vi "Acquire and Log Data - Config .vi"(5 "FPGA VI Reference":T5, 7 "Total Buffer Size":i32, 8 "error in (no error)":errorcluster, 9 "Number of Blocks Saved in":i32, 10 "Acquisition Data v1":T1={"Data Rate"=1, "Samples per Read"=0, "Number of Reads to Save"=0, "Data File Name"="", "TDMS Properties"=[], "Number of Channels"=4, "Channel Scale Array"=[0.0, 0.0, 0.0, 0.0, 0.0, 0.0, 0.0, 0.0, 0.0, 0.0, 0.0, 0.0, 0.0, 0.0, 0.0, 0.0, 0.0, 0.0, 0.0, 0.0, 0.0, 0.0, 0.0, 0.0], "Channel Names"=[], "Trigger - RMS Value"=0.0, "Trigger - Channel"=0, "Trigger - Time (Minute)"=0, "Input Configuration"=0} {"Input Configuration" items=["AC Coupled", "DC Coupled", "IEPE AC Coupled"]; "Data Rate" items=["51.200 kS/s (NI 9234)"=1, "25.600 kS/s (NI 9234)"=2, "17.067 kS/s (NI 9234)"=3, "12.800 kS/s (NI 9234)"=4, "10.240 kS/s (NI 9234)"=5, "8.533 kS/s (NI 9234)"=6, "7.314 kS/s (NI 9234)"=7, "6.400 kS/s (NI 9234)"=8, "5.689 kS/s (NI 9234)"=9, "5.120 kS/s (NI 9234)"=10, "4.654 kS/s (NI 9234)"=11, "4.267 kS/s (NI 9234)"=12, "3.938 kS/s (NI 9234)"=13, "3.657 kS/s (NI 9234)"=14, "3.413 kS/s (NI 9234)"=15, "3.200 kS/s (NI 9234)"=16, "3.012 kS/s (NI 9234)"=17, "2.845 kS/s (NI 9234)"=18, "2.695 kS/s (NI 9234)"=19, "2.560 kS/s (NI 9234)"=20, "2.438 kS/s (NI 9234)"=21, "2.328 kS/s (NI 9234)"=22, "2.226 kS/s (NI 9234)"=23, "2.133 kS/s (NI 9234)"=24, "2.048 kS/s (NI 9234)"=25, "1.969 kS/s (NI 9234)"=26, "1.896 kS/s (NI 9234)"=27, "1.829 kS/s (NI 9234)"=28, "1.765 kS/s (NI 9234)"=29, "1.707 kS/s (NI 9234)"=30, "1.652 kS/s (NI 9234)"=31]}, 11 "TDMS File Reference":refnum<k34>) -> (0 "error out":errorcluster, 1 "Number of Blocks Saved out":i32, 3 "Logging Complete?":bool)   [LabVIEW 2015]
doc: "Reads waveform data from the DMA FIFO."
uses:
  controls/FPGA VI Reference.ctl
  controls/Acquisition and Logging Configuration_v1.ctl
  <vilib>/LabVIEW Targets/FPGA/cRIO/shared/nicrio_ModuleControls/nicrio_cRIO-9234_DataRatesRing2.ctl
  controls/TDMS Properties.ctl
  <vilib>/LabVIEW Targets/FPGA/cRIO/shared/nicrio_ModuleControls/nicrio_cRIO-9234_ConfigModeRing.ctl
  <vilib>/Analysis/5stat.llb/RMS (DBL).vi
  Globals/Global - Monitoring Variables.vi
  <vilib>/Analysis/NI_AALPro.lvlib
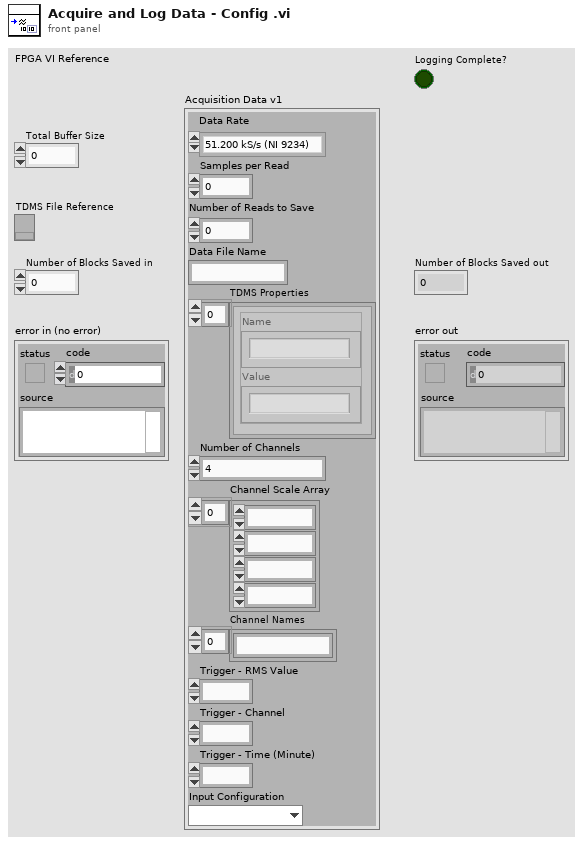
[diagram p1: front panel]
types:
  T1 = typedef "Acquisition and Logging Configuration_v1.ctl" = cluster{"Data Rate":T2, "Samples per Read":i32, "Number of Reads to Save":i32, "Data File Name":string, "TDMS Properties":T3[], "Number of Channels":i32, "Channel Scale Array":fxp<+,24,12>[], "Channel Names":string[], "Trigger - RMS Value":dbl, "Trigger - Channel":i32, "Trigger - Time (Minute)":i32, "Input Configuration":T4}
  T2 = typedef "nicrio_cRIO-9234_DataRatesRing2.ctl" = u8
  T3 = typedef "TDMS Properties.ctl" = cluster{"Name":string, "Value":string}
  T4 = typedef "nicrio_cRIO-9234_ConfigModeRing.ctl" = u8
  T5 = typedef "FPGA VI Reference.ctl" = refnum<k20>
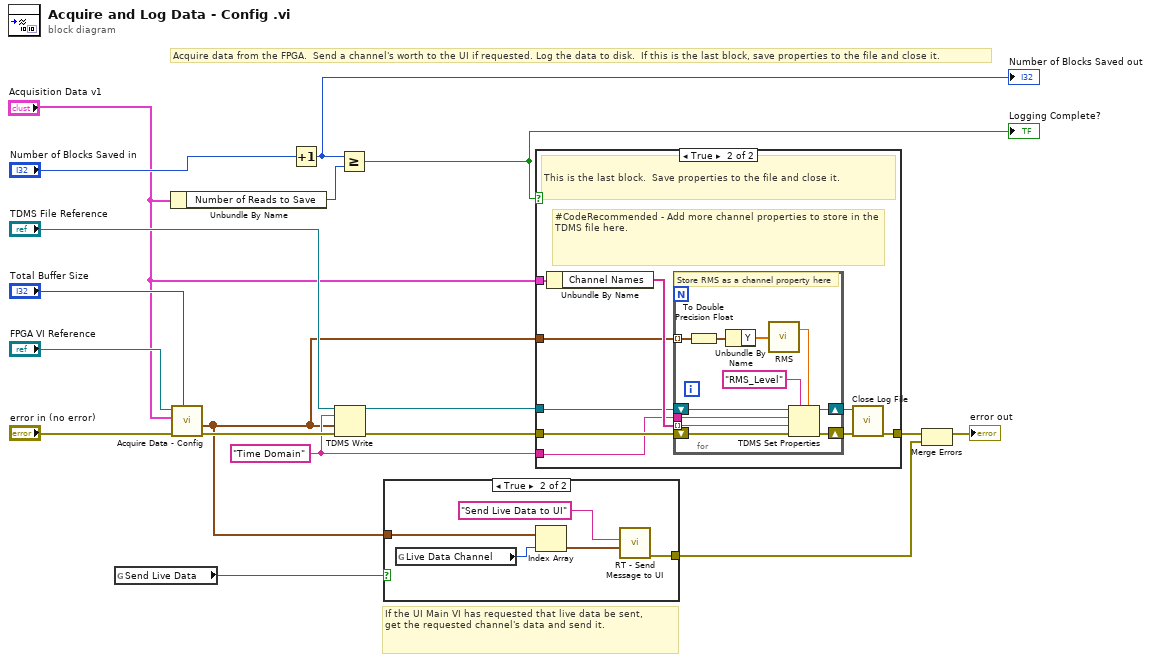
[diagram p0: block diagram]
diagram:
  w6 = "Time Domain" ("group name in (Untitled)")
  # "Acquire data from the FPGA.  Send a channel's worth to the UI if requested. Log the data to disk.  If this is the last block, save properties to the file and close it."
  # "If the UI Main VI has requested that live data be sent,\nget the requested channel's data and send it."
  n1 = global read "Global - Monitoring Variables.vi" "Send Live Data"() -> (w4:bool)
  n2 = Unbundle By Name("Acquisition Data v1") -> ("Number of Reads to Save"=w11:i32)
  n3 = call "Acquire Data - Config.vi"("Total Buffer Size"="Total Buffer Size", "error in (no error)"="error in (no error)", "Acquisition Data v1"="Acquisition Data v1", "FPGA VI Reference"="FPGA VI Reference") -> ("error out"=w15:errorcluster, "Waveform Data"=w3:waveform(sgl)[])  [unwired: 6 in]
  n4 = Increment(x="Number of Blocks Saved in") -> (x+1=w12:i32)
  "Number of Blocks Saved out" <- w12
  n5 = TDMS Write(0:"TDMS File Reference", 5:w6, 9:w3, 11:w15) -> (4:w9:refnum<k34>, 15:w8:errorcluster)  [unwired: 2 in, 2 out]
  n6 = Greater Or Equal?(x=w12, y=w11) -> (x >= y?=w10:bool)
  "Logging Complete?" <- w10
  n7 = case shown="True" w4 {
    tunnel: w3 -> [_ w23]
    tunnel: [_ w20] -> w2
    frame False {
    }
    frame True {
      n8 = global read "Global - Monitoring Variables.vi" "Live Data Channel"() -> (w22:u32)
      n9 = Index Array(array=w23, index=w22) -> (element=w21:waveform(sgl))
      n10 = call "RT - Send Message to UI.vi"("Message Data"=w21, "Message"="Send Live Data to UI" ("group name in (Untitled)")) -> ("error out"=w20:errorcluster)  [unwired: 9 in]
    }
  }
  n11 = case shown="True" w10 {
    tunnel: w9 -> [_ w29]
    tunnel: w8 -> [w24 w32]
    tunnel: [w24 w25] -> w7
    tunnel: "Acquisition Data v1" -> [_ w33]
    tunnel: w6 -> [_ w28]
    tunnel: w3 -> [_ w27]
    frame False {
      # "Do not finish the file.  This is not the last block."
    }
    frame True {
      # "#CodeRecommended - Add more channel properties to store in the TDMS file here."
      # "This is the last block.  Save properties to the file and close it."
      n12 = Unbundle By Name(w33) -> ("Channel Names"=w30:string[])
      n13 = for {
        tunnel: w28 -> [w41]
        shift-right: [w43] -> w31
        shift-left: w32 -> [w42]
        tunnel: w30 -> [w40] mode=indexing
        tunnel: w27 -> [w38] mode=indexing
        shift-right: [w35] -> w26
        shift-left: w29 -> [w44]
        # "Store RMS as a channel property here"
        n14 = To Double Precision Float(number=w38) -> (double precision float=w39:waveform(dbl))
        n15 = Unbundle By Name(w39) -> ("Y"=w34:dbl[])
        n16 = call-poly <vilib>:"RMS.vi"("X"=w34) -> ("rms value"=w37:dbl)  [unwired: 1 out]
        n17 = TDMS Set Properties(5:w37, 7:"RMS_Level" ("property names"), 8:w42, 9:w40, 10:w41, 11:w44) -> (0:w43:errorcluster, 3:w35:refnum<k34>)  [unwired: 2 out]
      }
      n18 = call "Close Log File.vi"("error in (no error)"=w31, "Log File"=w26) -> ("error out"=w25:errorcluster)  [unwired: 9 in]
    }
  }
  n19 = Merge Errors(w7, w2) -> (→"error out":errorcluster)
